vi "ReverseColumns.vi"(3 "output array 2":T1(array[cluster])) -> (1 "transposed array":T1(array[cluster]))   [LabVIEW 2015]
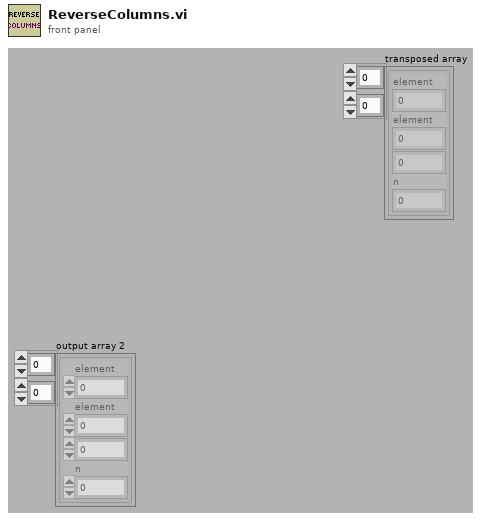
[diagram p1: front panel]
types:
  T1 = cluster{"element":u16, "element":u16, u16, "n":u16}[][]
  T2 = cluster{"element":u16, "element":u16, u16, "n":u16}[]
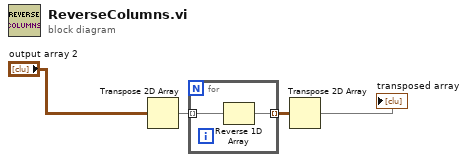
[diagram p0: block diagram]
diagram:
  n1 = Transpose 2D Array(2D array="output array 2") -> (transposed array=w3:T1)
  n2 = for {
    tunnel: w3 -> [w6] mode=indexing
    tunnel: [w5] -> w4 mode=indexing
    n3 = Reverse 1D Array(array=w6) -> (reversed array=w5:T2)
  }
  n4 = Transpose 2D Array(2D array=w4) -> (transposed array=→"transposed array":T1)
